vi "TURCK GUI TestPanel DXP.vi"() -> ()   [LabVIEW 2021]
doc: "Example for reading and writing Values for the TBEN-S1-8DXP module from Turck"
uses:
  KH TURCK ETHERNETIP TDefCluster TBEN-S1-8DXP Input Values.ctl
  KH TURCK ETHERNETIP TDefCluster TBEN-S1-8DXP Output Values.ctl
  KH EthernetIP 17.19/KH_EthernetIP_Globals.vi
panel:
  in  "Latch Reset":bool[](array[boolean])
  out "TBEN-S1-8DXP Input Values":T1
  out "DI":bool[](array[boolean])
  in  "DO":bool[](array[boolean])=[FALSE, FALSE, FALSE, FALSE]
  out "error out":errorcluster
  in  "Exit":bool
  # "- Before starting the VI your PC has to be in the same subnet as the modules\n- Channel 1-4 is configured as digital input\n- Channel 5-8 is configured as digital output"
  # "Kirschenhofer Maschinen GmbH\nRömerstraße 35, 89278 Nersingen-Straß\ninfo@kirschenhofer-gmbh.de"
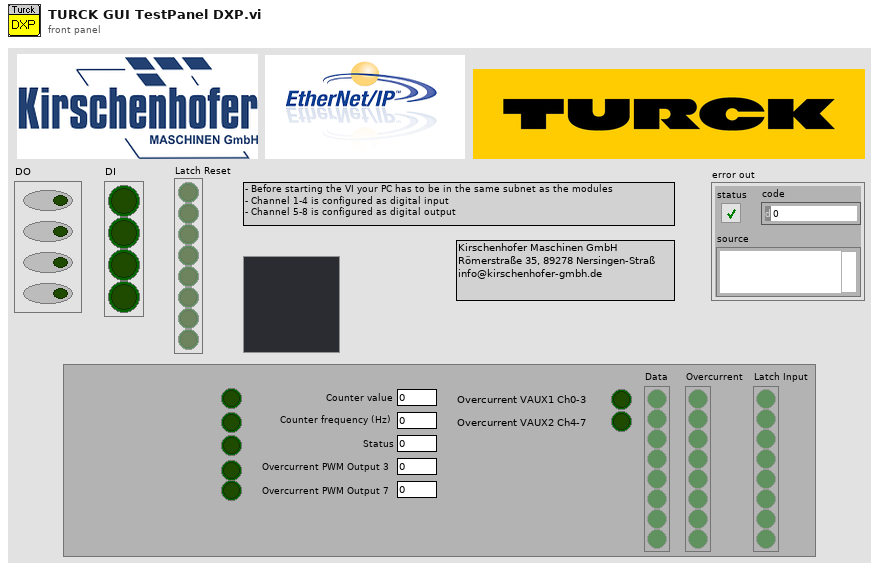
[diagram p1: front panel]
types:
  T1 = typedef "KH TURCK ETHERNETIP TDefCluster TBEN-S1-8DXP Input Values.ctl" = cluster{"Data":bool[], "Overcurrent":bool[], "Overcurrent VAUX1 Ch0-3":bool, "Overcurrent VAUX2 Ch4-7":bool, "Latch Input":bool[], "Counter value":u32, "Counter frequency (Hz)":u16, "Status":u8, "Overcurrent PWM Output 3":u8, "Overcurrent PWM Output 7":u8, "Module Diagnostics Available":bool, "INFO: ARGEE Project Running":bool, "Undervoltage V2":bool, "Undervoltage V1":bool, "Force Mode Enabled":bool}
  T2 = typedef "KH TURCK ETHERNETIP TDefCluster TBEN-S1-8DXP Output Values.ctl" = cluster{"Output Values":bool[], "Latch Resets":bool[], "Counter Reset":bool, "Duty Cycle Dig 3":u8, "Duty Cycle Dig 7":u8}
  T3 = cluster{"ItemCount":u16, "AdressItem":cluster{"TypeID":u16, "Length":u16, "Data":cluster{"ConnectionIdentifier":u32, "SequenceNumber":u32}}, "DataItem":cluster{"TypeID":u16, "Length":u16, "Data":u8[], "Sequence Count":u16}}
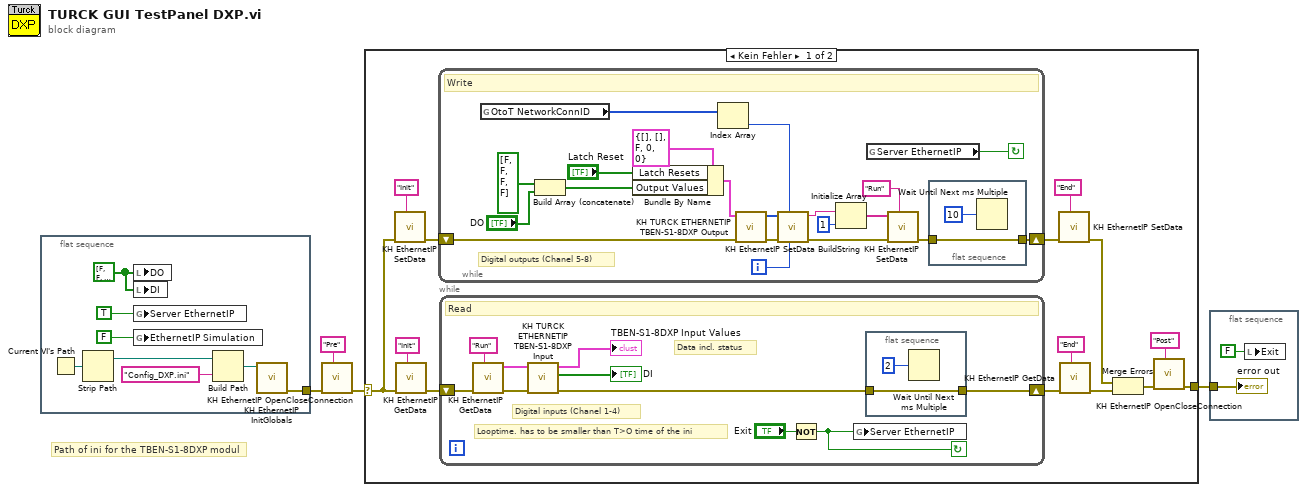
[diagram p0: block diagram]
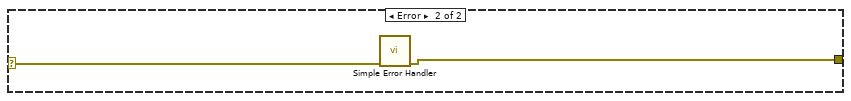
[diagram p2: hidden frame]
diagram:
  # "Path of ini for the TBEN-S1-8DXP modul"
  n1 = flat-sequence {
    tunnel: [w12] -> w3
    frame #0 {
      w10 = bool[] [FALSE, FALSE, FALSE, FALSE] ("DO")
      n2 = Current VI's Path() -> (path=w9:path)
      n3 = Strip Path(path=w9) -> (stripped path=w8:path)  [unwired: 1 out]
      n4 = local write "DO"(w10) -> ()
      n5 = local write "DI"(w10) -> ()
      n6 = global write "KH_EthernetIP_Globals.vi" "Server EthernetIP"(TRUE ("Server EthernetIP")) -> ()
      n7 = global write "KH_EthernetIP_Globals.vi" "EthernetIP Simulation"(FALSE ("EthernetIP Simulation")) -> ()
      n8 = Build Path(base path=w8, name or relative path="Config_DXP.ini") -> (appended path=w6:path)
      n9 = call "KH EthernetIP InitGlobals.vi"("Config File"=w6) -> ("err out"=w12:errorcluster)  [unwired: 10 in]
    }
  }
  n10 = call "KH EthernetIP OpenCloseConnection.vi"("Function"="Pre", "error in"=w3) -> ("error out"=w1:errorcluster)  [unwired: 9 in]
  n11 = case shown="Kein Fehler" w1 {
    selector: w1 -> [w13 w62]
    tunnel: [w14 w61] -> w2
    frame No Error {
      n12 = call "KH EthernetIP SetData.vi"("Function"="Init", "error in"=w13) -> ("error out"=w16:errorcluster)  [unwired: 7 in, 2 out]
      n13 = call "KH EthernetIP GetData.vi"("Function"="Init", "error in"=w13) -> ("error out"=w26:errorcluster)  [unwired: 8 in, 1 out]
      n14 = while {
        shift-right: [w44] -> w17
        shift-left: w16 -> [w32]
        i -> [w33]
        stop <- w43 continue-if-true
        # "Digital outputs (Chanel 5-8)"
        # "Write"
        n15 = global read "KH_EthernetIP_Globals.vi" "OtoT NetworkConnID"() -> (w28:u32[])
        n16 = Build Array (concatenate)(bool[] [FALSE, FALSE, FALSE, FALSE] ("DataDXPout"), "DO") -> (w30:bool[])
        n17 = Bundle By Name(cluster=T2 {"Output Values"=[], "Latch Resets"=[], "Counter Reset"=FALSE, "Duty Cycle Dig 3"=0, "Duty Cycle Dig 7"=0} ("TBEN-S1-8DXP Output Values"), "Latch Resets"="Latch Reset", "Output Values"=w30) -> (w40:T2)
        n18 = Index Array(array=w28) -> (element=w27:u32)  [unwired: 1 in]
        n19 = call "KH TURCK ETHERNETIP TBEN-S1-8DXP Output.vi"("error in"=w32, "TBEN-S1-8DXP Output Values"=w40) -> ("error out"=w39:errorcluster, "Output Data"=w38:u8[])  [unwired: 8 in]
        n20 = call "KH EthernetIP SetData BuildString.vi"("LoopIndex"=w33, "OtoT NetworkConnID"=w27, "error in"=w39, "Output Data"=w38) -> ("error out"=w31:errorcluster, "DataString"=w37:string)  [unwired: 6 in]
        n21 = Initialize Array(w37, 1 ("dimension size")) -> (w34:string[])
        n22 = global read "KH_EthernetIP_Globals.vi" "Server EthernetIP"() -> (w43:bool)
        n23 = call "KH EthernetIP SetData.vi"("Function"="Run", "error in"=w31, "Data Strings"=w34) -> ("error out"=w45:errorcluster)  [unwired: 6 in, 2 out]
        n24 = flat-sequence {
          tunnel: w45 -> [w47]
          tunnel: [w47] -> w44
          frame #0 {
            n25 = Wait Until Next ms Multiple(millisecond multiple=u32 10) -> ()  [unwired: 1 out]
          }
        }
      }
      n26 = while {
        shift-right: [w56] -> w24
        shift-left: w26 -> [w58]
        stop <- w49 continue-if-true
        # "Data incl. status"
        # "Looptime. has to be smaller than T>O time of the ini"
        # "Digital inputs (Chanel 1-4)"
        # "Read"
        n27 = call "KH EthernetIP GetData.vi"("Function"="Run", "error in"=w58) -> ("error out"=w52:errorcluster, "Response Data"=w54:T3)  [unwired: 8 in]
        n28 = call "KH TURCK ETHERNETIP TBEN-S1-8DXP Input.vi"("error in"=w52, "Response Data"=w54) -> ("error out"=w51:errorcluster, "DataDXP"=→"DI":bool[], "TBEN-S1-8DXP Input Values"=→"TBEN-S1-8DXP Input Values":T1)  [unwired: 7 in]
        n29 = Not(x="Exit") -> (.not. x?=w49:bool)
        n30 = global write "KH_EthernetIP_Globals.vi" "Server EthernetIP"(w49) -> ()
        n31 = flat-sequence {
          tunnel: w51 -> [w59]
          tunnel: [w59] -> w56
          frame #0 {
            n32 = Wait Until Next ms Multiple(millisecond multiple=u32 2) -> ()  [unwired: 1 out]
          }
        }
      }
      n33 = call "KH EthernetIP SetData.vi"("Function"="End", "error in"=w17) -> ("error out"=w21:errorcluster)  [unwired: 7 in, 2 out]
      n34 = call "KH EthernetIP GetData.vi"("Function"="End", "error in"=w24) -> ("error out"=w19:errorcluster)  [unwired: 8 in, 1 out]
      n35 = Merge Errors(w21, w19) -> (w20:errorcluster)
      n36 = call "KH EthernetIP OpenCloseConnection.vi"("Function"="Post", "error in"=w20) -> ("error out"=w14:errorcluster)  [unwired: 9 in]
    }
    frame Error {
      n37 = call <vilib>:"Simple Error Handler.vi"("error in (no error)"=w62) -> ("error out"=w61:errorcluster)  [unwired: 4 in, 4 out]
    }
  }
  n38 = flat-sequence {
    tunnel: w2 -> [w63]
    frame #0 {
      n39 = local write "Exit"(FALSE ("Exit")) -> ()
      "error out" <- w63
    }
  }
